vi "recording and saving.vi"() -> ()   [LabVIEW 2017]
uses:
  <vilib>/sound2/lvsound2.llb/Sampling Mode.ctl
  <vilib>/sound2/lvsound2.llb/Sound Data Format.ctl
  <vilib>/sound2/lvsound2.llb/Sound File Write Open.vi
  <vilib>/sound2/lvsound2.llb/Sound Input Read (DBL).vi
  <vilib>/sound2/lvsound2.llb/Sound File Write (DBL).vi
  <vilib>/measure/mascope.llb/Cycle Average and RMS N chan.vi
  <vilib>/Waveform/WDTFileIO.llb/Export Waveforms To Spreadsheet File (1D).vi
  <vilib>/measure/NI_MAPro.lvlib
panel:
  out "cycle average":dbl[](array[numeric]) format="%.2p"
  out "cycle RMS":dbl[](array[numeric]) format="%.2p"
  in  "excel file":path
  in  "main signal":path
  out "main signal":waveform(dbl)[](graph)
  in  "stop":bool
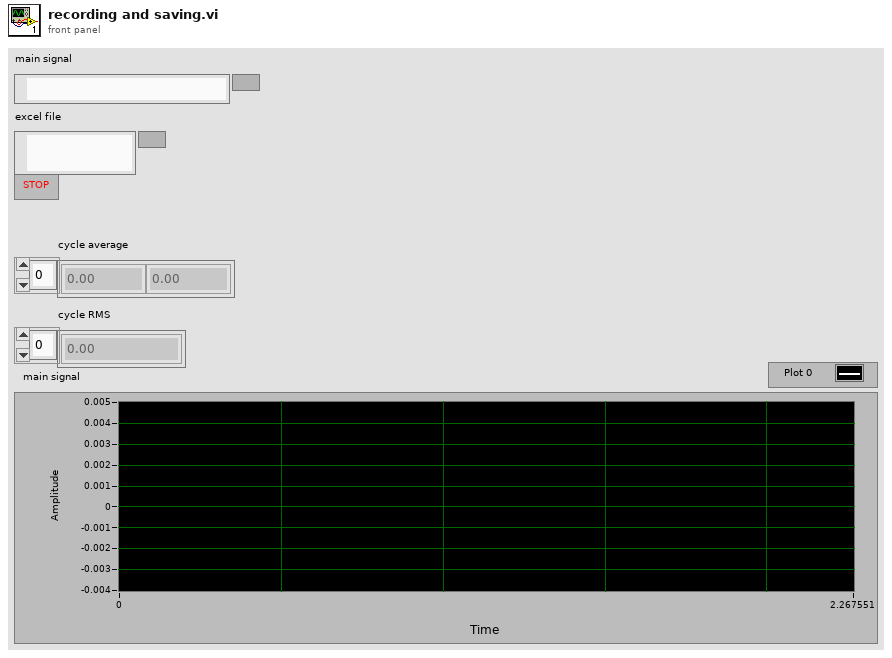
[diagram p1: front panel]
types:
  T1 = typedef "Sound Data Format.ctl" = cluster{"sample rate (S/s)":dbl, "number of channels":i32, "bits per sample":i32}
  T2 = typedef "Sampling Mode.ctl" = i32
  T3 = typedef "Sound File Refnum.ctl" = refnum<file>
  T4 = typedef "Sound Input Task ID.ctl" = u32
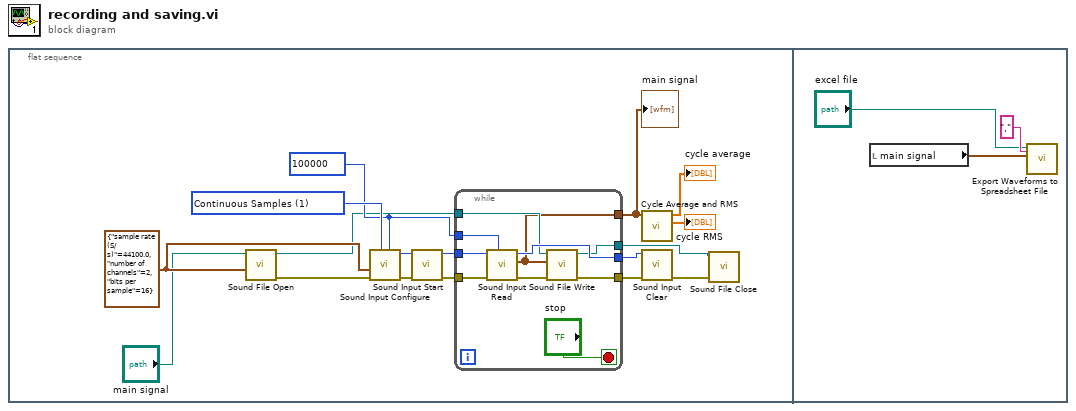
[diagram p0: block diagram]
diagram:
  n1 = flat-sequence {
    frame #0 {
      w10 = T1 {"sample rate (S/s)"=44100.0, "number of channels"=2, "bits per sample"=16} ("sound format")
      w16 = 100000 ("number of samples/ch")
      w17 = T2 1 items=["Finite Samples", "Continuous Samples"] ("sample mode")
      n2 = call-poly <vilib>:"Sound File Open.vi"("sound format"=w10, "path"="main signal") -> ("error out"=w7:errorcluster, "sound file refnum"=w9:T3)  [unwired: 8 in]
      n3 = call <vilib>:"Sound Input Configure.vi"("number of samples/ch"=w16, "sample mode"=w17, "error in (no error)"=w7, "sound format"=w10) -> ("error out"=w13:errorcluster, "task ID"=w14:T4)  [unwired: 6 in]
      n4 = call <vilib>:"Sound Input Start.vi"("error in (no error)"=w13, "task ID"=w14) -> ("error out"=w12:errorcluster, "task ID out"=w11:T4)  [unwired: 8 in]
      n5 = while {
        tunnel: w11 -> [w27]
        tunnel: w12 -> [w24]
        tunnel: w16 -> [w26]
        tunnel: [w25] -> w15
        tunnel: [w23] -> w2
        tunnel: w9 -> [w22]
        tunnel: [w19] -> w6
        tunnel: [w18] -> w5
        stop <- "stop" stop-if-true
        n6 = call-poly <vilib>:"Sound Input Read.vi"("number of samples/ch"=w26, "error in (no error)"=w24, "task ID"=w27) -> ("error out"=w20:errorcluster, "data"=w18:waveform(dbl)[], "task ID out"=w25:T4)  [unwired: 6 in]
        n7 = call-poly <vilib>:"Sound File Write.vi"("error in (no error)"=w20, "data"=w18, "sound file refnum"=w22) -> ("error out"=w19:errorcluster, "sound file refnum out"=w23:T3)  [unwired: 7 in]
      }
      "main signal" <- w5
      n8 = call-poly <vilib>:"Cycle Average and RMS.vi"("signal(s) in"=w5) -> ("cycle RMS"=→"cycle RMS":dbl[], "cycle average"=→"cycle average":dbl[])  [unwired: 7 in, 2 out]
      n9 = call <vilib>:"Sound Input Clear.vi"("error in (no error)"=w6, "task ID"=w15) -> ("error out"=w1:errorcluster)  [unwired: 9 in]
      n10 = call <vilib>:"Sound File Close.vi"("error in (no error)"=w1, "sound file refnum"=w2) -> ()  [unwired: 9 in, 1 out]
    }
    frame #1 {
      n11 = local read "main signal"() -> (w30:waveform(dbl)[])
      n12 = call-poly <vilib>:"Export Waveforms to Spreadsheet File.vi"("delimiter (Tab)"=",", "waveforms"=w30, "file path (dialog if empty)"="excel file") -> ()  [unwired: 7 in, 2 out]
    }
  }
